vi "Read Parameter.vi"(8 "error in (no error)":errorcluster, 11 "SqlMapper in":refnum<class "DapperMapper.lvclass">) -> (0 "error out":errorcluster, 2 "DynamicParameters out":refnum<class "DynamicParameters.lvclass">, 3 "SqlMapper out":refnum<class "DapperMapper.lvclass">)   [LabVIEW 2020, in "ORM_Dapper.lvlib" / "DapperMapper.lvclass"]
uses:
  DapperMapper.lvclass
  <vilib>/Viviota/shared/ORM.lvlibp/ORM/DynamicParameters/DynamicParameters.lvclass
  DapperParameters/DapperParameters.lvclass
  C:/Program Files/National Instruments/LabVIEW 2020/vi.lib/Viviota/shared/ORM.lvlibp/ORM/DynamicParameters/DynamicParameters.lvclass
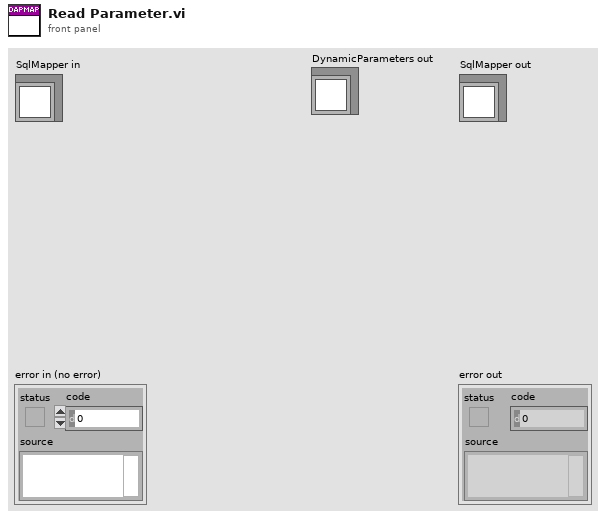
[diagram p1: front panel]
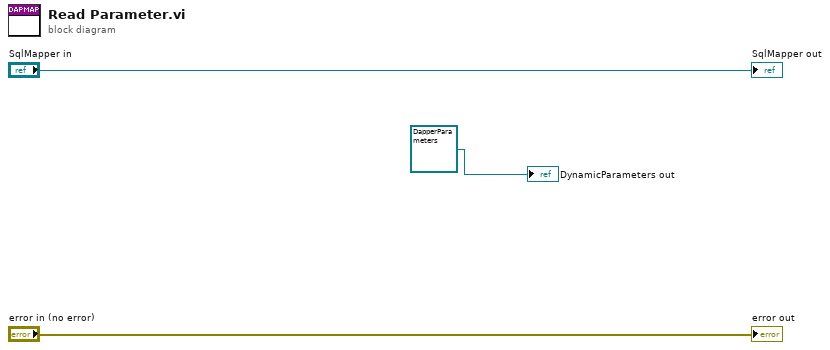
[diagram p0: block diagram]
diagram:
  "error out" <- "error in (no error)"
  "SqlMapper out" <- "SqlMapper in"
  "DynamicParameters out" <- refnum<class "DapperParameters.lvclass"> refnum ("Dapper.lvlib:DynamicParameters")
